vi "CoboltLaser_SetpointSet.vi"(0 "ComPort":refnum<visa-resource-name>, 5 "CheckResponse":bool=TRUE, 7 "Setpoint_Un":dbl format="%.3g", 9 "Mode":T1 caption="Laser Mode", 11 "ErrorIn":errorcluster, 12 "CurrentModLow":bool) -> (4 "ComPortOut":refnum<visa-resource-name>, 6 "Setpoint_Un":dbl format="%.3g", 8 "Setpoint_Pc":dbl, 10 "Response":string, 13 "MaxSetpoint":dbl, 14 "ResponseOK":bool, 15 "ErrorOut":errorcluster)   [LabVIEW 2019]
doc: "Use this template to build a VI to use as a subVI."
uses:
  Programmes Labview/LabscanV1A/DevicesClass/InstrumentsClass/CoboltMLD/CoboltModes.ctl
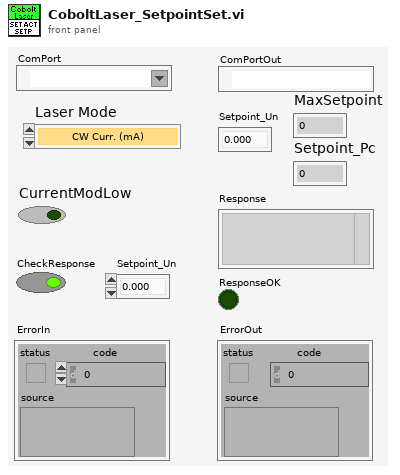
[diagram p1: front panel]
types:
  T1 = typedef "CoboltModes.ctl" = enum16{"CW Curr. (mA)", "CW Pow. (mW)", "Curr. Mod. (mA)", "Pow. Mod. (mW)"}
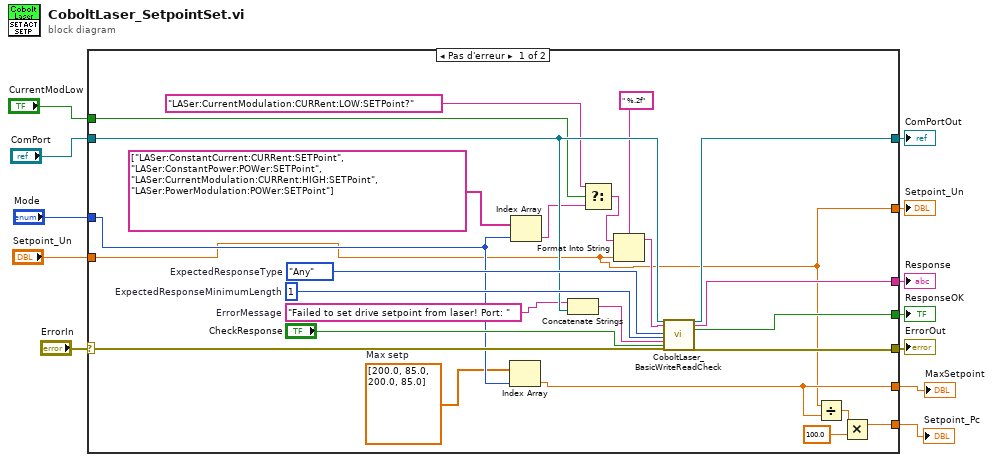
[diagram p0: block diagram]
diagram:
  n1 = case shown="Pas d'erreur" "ErrorIn" {
    selector: "ErrorIn" -> [w37 w39]
    tunnel: [w36 w39] -> w11
    tunnel: "ComPort" -> [w31 w38]
    tunnel: [w30 w38] -> w9
    tunnel: [w13 _] -> w8
    tunnel: [w29 _] -> w7
    tunnel: [w28 _] -> w6
    tunnel: "Mode" -> [w23 _]
    tunnel: "CurrentModLow" -> [w24 _]
    tunnel: [w21 _] -> w3
    tunnel: [w19 _] -> w2
    tunnel: "Setpoint_Un" -> [w13 _]
    frame No Error {
      w22 = dbl[] [200.0, 85.0, 200.0, 85.0]  # Max setp
      w34 = 1  # ExpectedResponseMinimumLength
      w35 = enum16{"Any", "Digits Only", "Non-Digits Only"}."Any"  # ExpectedResponseType
      w14 = "Failed to set drive setpoint from laser! Port: "  # ErrorMessage
      n2 = Index Array(array=w22, index=w23) -> (element=w21:dbl)
      n3 = Index Array(array=string[] ["LASer:ConstantCurrent:CURRent:SETPoint", "LASer:ConstantPower:POWer:SETPoint", "LASer:CurrentModulation:CURRent:HIGH:SETPoint", "LASer:PowerModulation:POWer:SETPoint"] ("tableau ajouté"), index=w23) -> (element=w26:string)
      n4 = Concatenate Strings(w14, w31) -> (w32:string)
      n5 = Select(t="LASer:CurrentModulation:CURRent:LOW:SETPoint?" ("Command"), s=w24, f=w26) -> (s? t:f=w17:string)
      n6 = Format Into String(format string=" %.2f" ("chaîne de format"), initial string=w17, w13) -> (resulting string=w15:string)  [unwired: 1 in, 1 out]
      n7 = call <userlib>:"CoboltLaser_BasicWriteReadCheck.vi"("ComPort"=w31, "Command"=w15, "ExpectedResponseType"=w35, "ExpectedResponseMinimumLength"=w34, "ErrorMessage"=w32, "GenerateError"="CheckResponse", "error in (no error)"=w37) -> ("ComPortOut"=w30:refnum<visa-resource-name>, "Response"=w29:string, "ResponseOK"=w28:bool, "error out"=w36:errorcluster)  [unwired: 17 in]
      n8 = Divide(x=w13, y=w21) -> (x/y=w20:dbl)
      n9 = Multiply(x=w20, y=100.0) -> (x*y=w19:dbl)
    }
    frame Error {
    }
  }
  "ErrorOut" <- w11
  "ComPortOut" <- w9
  "Response" <- w7
  "ResponseOK" <- w6
  "Setpoint_Un" <- w8
  "MaxSetpoint" <- w3
  "Setpoint_Pc" <- w2
